vi "EnqueueMulitpleMainController.vi"(6 "timeout in ms (-1)":i32=-1, 8 "error in (no error)":errorcluster, 9 "Data":variant[](array[variant]), 10 "Messages":T1[](array[typedef]), 11 "MainQueue":refnum<queue>) -> (0 "error out":errorcluster, 1 "timed out?":bool, 3 "MainQueue out":refnum<queue>)   [LabVIEW 2019, in "MainController.lvlib"]
uses:
  MainController.lvlib
  Cluster - MainControllerMessage.ctl
  Enum - MainState.ctl
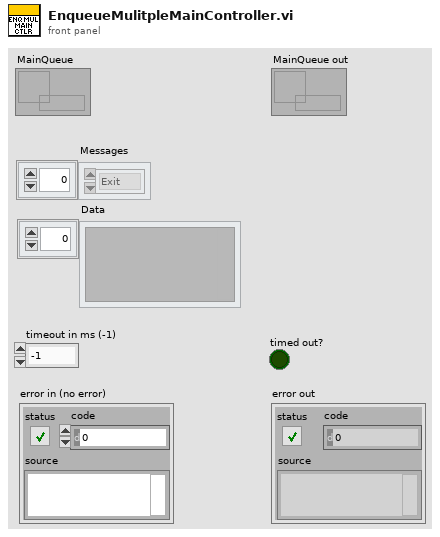
[diagram p1: front panel]
types:
  T1 = typedef "MainController.lvlib/Enum - MainState.ctl" = enum16{"Initialize", "InitUIRefs", "LaunchSettings", "LaunchAutoMode", "LaunchManualMode", "LaunchTestReport", "ConnectHardware", "DisconnectHardware", "HiliteNavItems", "StartAutoMode", "PauseAutoMode", "StopAutoMode", "ShowFlyout", "HideFlyout", "BroadcastSettings", "PickupTestSettings", "BroadcastHW", "AutoTestDone", "DAQStatus", "UpdateCommandBar", "Error", "RecieveError", "Exit"}
  T2 = typedef "MainController.lvlib/Cluster - MainControllerMessage.ctl" = cluster{"Message":T1, "Data":variant}
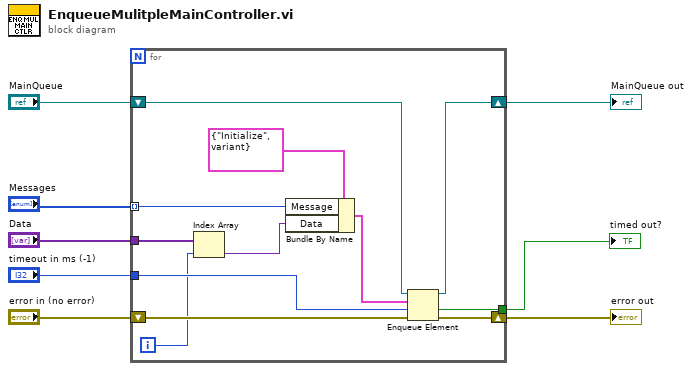
[diagram p0: block diagram]
diagram:
  n1 = for {
    tunnel: "timeout in ms (-1)" -> [w17]
    tunnel: [w13] -> w3
    tunnel: "Data" -> [w11]
    tunnel: "Messages" -> [w12] mode=indexing
    shift-right: [w16] -> w4
    shift-left: "error in (no error)" -> [w20]
    shift-right: [w19] -> w7
    shift-left: "MainQueue" -> [w18]
    i -> [w10]
    n2 = Index Array(array=w11, index=w10) -> (element=w9:variant)
    n3 = Bundle By Name(cluster=T2 {"Message"=enum."Initialize", "Data"=variant} ("Message"), "Message"=w12, "Data"=w9) -> (w14:T2)
    n4 = Enqueue Element(queue=w18, element=w14, timeout in ms (-1)=w17, error in (no error)=w20) -> (queue out=w19:refnum<queue>, timed out?=w13:bool, error out=w16:errorcluster)
  }
  "error out" <- w4
  "MainQueue out" <- w7
  "timed out?" <- w3
